vi "Test Ultrasonic.vi"() -> ()   [LabVIEW 2013]
uses:
  <vilib>/Rock Robotics/SystemInterfaces/Typedef/FPGA_TypedefDigitalModule.ctl
panel:
  out "Distance":dbl
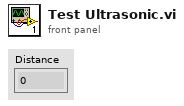
[diagram p1: front panel]
types:
  T1 = typedef "FPGA_TypedefDigitalModule.ctl" = enum16{"Digital Module 1", "Digital Module 2"}
  T2 = typedef "WPI_I2CDevRef.ctl" = cluster{"DevStatus":errorcluster, "Digital Module":T1, "Device Address":u8}
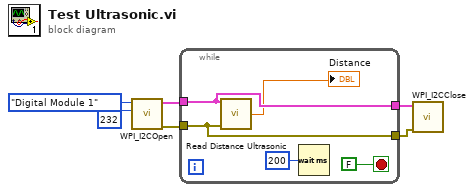
[diagram p0: block diagram]
diagram:
  n1 = call <vilib>:"WPI_I2COpen.vi"("Device Address"=u8 232, "Digital Module (Module 1)"=FPGA_TypedefDigitalModule."Digital Module 1") -> ("error out"=w3:errorcluster, "I2CDevRef"=w4:T2)  [unwired: 8 in]
  n2 = while {
    tunnel: w4 -> [w9]
    tunnel: w3 -> [w8]
    tunnel: [w9] -> w2
    tunnel: [w8] -> w1
    stop <- FALSE stop-if-true
    n3 = call "Read Distance Ultrasonic.vi"("error out"=w8, "I2CDevRef"=w9) -> ("Inch"=→"Distance":dbl)
    n4 = Wait (ms)(milliseconds to wait=u32 200) -> ()  [unwired: 1 out]
  }
  n5 = call <vilib>:"WPI_I2CClose.vi"("error in (no error)"=w1, "I2CDevRef"=w2) -> ()  [unwired: 9 in, 1 out]
